vi "DI Scope Run.vi"(8 "error in":errorcluster, 11 "RT Data In":refnum<class "DCM-NIVS-RT.lvclass">) -> (0 "error out":errorcluster, 3 "RT Data Out":refnum<class "DCM-NIVS-RT.lvclass">)   [LabVIEW 2016, in "DCM Engine.lvlib"]
uses:
  DCM Engine.lvlib
  Classes/DCM-NIVS-RT/DCM-NIVS-RT.lvclass
  Classes/DCM-NIVS-RT/CompiledData Read.vi
  Classes/DCM-NIVS-RT/DCM Ref Read.vi
  Classes/DCM-NIVS-RT/Device Inputs Read.vi
  Classes/DCM-NIVS-RT/Device Outputs Read.vi
  Classes/DCM-NIVS-RT/CompiledData Write.vi
  Classes/DCM-NIVS-RT/Device Outputs Write.vi
  <vilib>/NI Veristand/Custom Device Waveform API/Multiple Waveforms Write (DBL)/Multiple Waveforms Write (DBL).lvclass
  Built/DCM Classes Packed/Pharlap/C/DCM-Classes.lvlibp/DCM/Rev0/RT/DCM - RT.lvclass
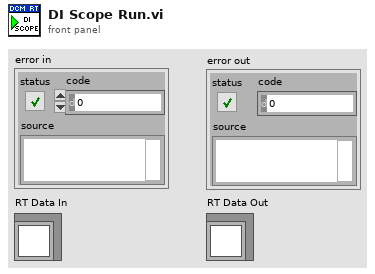
[diagram p1: front panel]
types:
  T1 = typedef "DCM Shared.lvlib/Compiled Data.ctl" = cluster{"Init":T2, "Cmd Status":T3, "Sys Status":T3, "EPTx RevA":T4, "DCM Core":T7, "DI-A Injection":T17, "DI-B Injection":T17, "DiffIO":T24, "HH Cmd":T27, "DI ADC":T29, "HH ADC":T31, "Digital Signals":T32, "Skip Fire":T33, "Knock":T35, "PBx":T36}
  T2 = typedef "DCM Shared.lvlib/Engine Init Data.ctl" = cluster{"Name":string, "RIO Address":string, "Bitfile Path RT":path, "Username":string, "Password":string, "Cmd CPU":i32, "Cmd Decimation":i32, "Cmd Priority":i32, "Sys CPU":i32, "Sys Decimation":i32, "Sys Priority":i32, "Input FIFO Size":i32, "Output FIFO Size":i32, "Compile Time":dbl}
  T3 = typedef "DCM Shared.lvlib/Engine Status.ctl" = cluster{"FIFO indexes":cluster{"code":i32, "loop duration":i32, "late count":i32}}
  T4 = typedef "DCM Shared.lvlib/EPTx RevA RT Data.ctl" = cluster{"FIFO Indexes":cluster{"Read":cluster{"Sync":i32, "CurrentCAD":i32, "Speed":i32, "Config":i32, "Rcvg Primary":i32, "Stall":i32, "Overflow Error":i32, "Ratio Error":i32, "Pattern Error":i32, "Aux Warning":i32, "Watchdog Error":i32, "Loading":i32}, "Write":cluster{"Reload EPTx":i32, "Sync Enable":i32, "Clear Errors":i32, "Sim Enable":i32, "Sim Speed":i32}}, "Settings":cluster{"EPTxConfigFilename":string, "EPTx Signal Select":cluster{"Primary":T5, "Aux 1":T5, "Aux 2":T5, "Aux 3":T5, "Aux 4":T5}, "FPGAFrequency":sgl, "StallSpeed":sgl, "EPTxFilters":T6, "History":u8}}
  T5 = typedef "DCM-Classes.lvlibp/DCM - FPGA.lvlib/Digital Channel.ctl" = enum8{"Unused", "User OS", "Diff IO 1", "Diff IO 2", "Diff IO 3", "Diff IO 4", "Diff IO 5", "Diff IO 6", "Diff IO 7", "Diff IO 8", "Aux 1", "Aux 2", "Aux 3", "Aux 4", "Aux 5", "Aux 6", "Aux 7", "Aux 8", "Aux 9", "Aux 10", "Aux 11", "Aux 12", "Aux 13", "Aux 14", "Aux 15", "Aux 16"}
  T6 = typedef "DCM-Classes.lvlibp/EPTx - RevA - RT.lvlib/EPTxFilters.ctl" = cluster{"Primary [s]":sgl, "Aux 1 [s]":sgl, "Aux 2 [s]":sgl, "Aux 3 [s]":sgl, "Aux 4 [s]":sgl}
  T7 = typedef "DCM Shared.lvlib/DCM Core.ctl" = cluster{"FIFO Indexes":cluster{"A Run State":i32, "B Run State":i32, "Read":cluster{"Status":T8, "A DI Faults":T9[], "B DI Faults":T9[], "HH Status":T10[]}, "Write":cluster{"A Config":cluster{"PowerSupplyEnable":i32, "InjectEnable":i32, "BoostVoltage":i32}, "B Config":cluster{"PowerSupplyEnable":i32, "InjectEnable":i32, "BoostVoltage":i32}, "HH Config":T11[], "System Settings":cluster{"MPRD":i32, "UserLED1":i32, "UserLED2":i32}, "A Fault Clear":cluster{"1":i32, "2":i32, "3":i32, "4":i32, "5":i32, "6":i32, "7":i32, "8":i32}, "B Fault Clear":cluster{"1":i32, "2":i32, "3":i32, "4":i32, "5":i32, "6":i32, "7":i32, "8":i32}}}, "Settings":cluster{"A Configuration":T12, "B Configuration":T12, "System Settings":T14}}
  T8 = typedef "DCM Shared.lvlib/System State Indexes.ctl" = cluster{"System ADC":cluster{"AI 1 [V]":i32, "AI 2 [V]":i32, "AI 3 [V]":i32, "AI 4 [V]":i32, "AI 5 [V]":i32, "AI 6 [V]":i32, "AI 7 [V]":i32, "AI 8 [V]":i32, "AI 9 [V]":i32, "AI 10 [V]":i32, "AI 11 [V]":i32, "AI 12 [V]":i32, "Temp HH 1-6 [C]":i32, "Temp HH 7-12 [C]":i32, "Temp DI A [C]":i32, "Temp DI Zener A [C]":i32, "Temp DI B [C]":i32, "Temp DI Zener B [C]":i32, "Temp CPU [C]":i32, "Temp Fan Intake [C]":i32, "Temp Secondary A [C]":i32, "Temp Primary A [C]":i32, "Temp Boost B [C]":i32, "Primary Range [V]":i32, "Primary A1A2 [V]":i32, "Primary A3A4 [V]":i32, "Primary B3B4 [V]":i32, "Primary B1B2 [V]":i32, "Secondary A1A2 [V]":i32, "Secondary A3A4 [V]":i32, "Secondary B3B4 [V]":i32, "Secondary B1B2 [V]":i32, "Ext HV A [V]":i32, "Ext HV B [V]":i32, "FET Driver [V]":i32, "Fan [V]":i32, "Battery [V]":i32, "DRVP [V]":i32, "Key [V]":i32, "DI Zener A [V]":i32, "DI Zener B [V]":i32, "Pump Zener A [V]":i32, "Pump Zener B [V]":i32, "MPRD [V]":i32}, "IO Lock":i32, "HH Mode Config Error":i32, "Fan Speed 1 [RPM]":i32, "Fan Speed 2 [RPM]":i32, "Firmware Major Rev":i32, "Firmware Minor Rev":i32, "Internal Fault":i32, "Fault Value":i32}
  T9 = typedef "DCM Shared.lvlib/DI Faults Indexes.ctl" = cluster{"HV Fault":i32, "LV Fault":i32, "LS Fault":i32, "MUX Fault":i32, "Open Warning":i32}
  T10 = typedef "DCM Shared.lvlib/HH Status Indexes.ctl" = cluster{"Current [A]":i32, "Config Error":i32, "Short Fault":i32, "Open Fault":i32, "Period Min [A]":i32, "Period Max [A]":i32, "Period Avg [A]":i32, "On Avg [A]":i32}
  T11 = typedef "DCM Shared.lvlib/HH Config Indexes.ctl" = cluster{"Mode":i32, "IO Lock State":i32, "Phase 1 FP":i32, "Fault Clear":i32, "ISeq":cluster{"Upper [A]":i32, "Lower [A]":i32, "Duration [s]":i32}[]}
  T12 = typedef "DCM - RT.lvclass/Configuration.ctl" = cluster{"Configuration":T13, "Power Supply Enable":bool, "Boost Voltage [V]":sgl, "Inject Enable":bool, "DI Zener Enable":bool, "DI Zener Voltage [V]":sgl, "Pump Zener Enable":bool, "Pump Zener Voltage [V]":sgl, "Boost Clamp [V]":sgl}
  T13 = typedef "DCM - FPGA.lvlib/DI - Bank Configuration.ctl" = enum8{"Solenoid Unipolar 4", "Solenoid Unipolar 7 (Muxed)", "Solenoid Unipolar 8 (Muxed)", "Solenoid Bipolar 2", "Solenoid Bipolar 3 (Muxed)", "Piezo Unipolar 2", "Piezo Unipolar 3 (Muxed)", "Piezo Unipolar 4 (Muxed)", "Piezo Bipolar 2", "Piezo Bipolar 3 (Muxed)"}
  T14 = typedef "DCM - RT.lvclass/System Settings.ctl" = cluster{"MPRD":bool, "IO Lock MPRD Disable":bool, "User LED 1":T15, "User LED 2":T15, "DI HS Fault Filter Time [s]":sgl, "Clamp Fault Filter Time [s]":sgl, "HH Shoot Through Time [s]":sgl, "HH ISeq Dur PS":T16, "HH Open Threshold [A]":sgl}
  T15 = typedef "DCM - RT.lvclass/User LED.ctl" = enum16{"Off", "Yellow", "Green"}
  T16 = typedef "DCM - RT - HH.lvlib/Duration Pre Scale.ctl" = u8
  T17 = typedef "DCM Shared.lvlib/DI.ctl" = cluster{"DI Command Enabled":bool, "Sync Pump Enabled":bool, "FIFO Indexes":cluster{"Write":cluster{"DI Command":T18[], "Pump Command":T18}}, "Settings":T19}
  T18 = typedef "DCM Shared.lvlib/DI Command Indexes.ctl" = cluster{"Mode":i32, "Digital Input":i32, "Default Profile Index":i32, "Cal Freq [Hz]":i32, "Cal Duration [s]":i32, "Cal Increment [s]":i32, "Cal Pulses":i32, "TMP Command Sequence":cluster{"Duration [s]":i32, "Level":i32, "Run/Stop":i32, "Profile Index":i32}[], "EPT TDC Offset [CAD]":i32, "EPT Window Start [DBTDC]":i32, "EPT Window End [DBTDC]":i32, "EPT Angles":cluster{"Enable":i32, "Timing [DBTDC]":i32, "Duration [s]":i32, "Profile Index":i32}[], "EPT Skip Fire":i32, "EPT Skip Index":i32, "EPT Precharge Duration [s]":i32, "EPT Precharge Profile Index":i32}
  T19 = typedef "DCM Shared.lvlib/DI Phase Outputs.ctl" = cluster{"Inj Phase Arrays":T20[][], "Pump Phase Array":T20[], "Pulsewidths [s]":sgl[][]}
  T20 = typedef "DCM - RT - DI.lvlib/Phase.ctl" = cluster{"Drive":T21, "Direction":bool, "Phase Step":T22, "Duration [s]":sgl, "Current High [A]":sgl, "Current Low [A]":sgl, "Voltage High [V]":sgl, "Voltage Low [V]":sgl, "Change":bool, "Current Control":T23, "Period [s]":sgl, "Pulse Width [s]":sgl, "Profile":u8, "Voltage Control":bool}
  T21 = typedef "DCM - FPGA.lvlib/DI - Drive State.ctl" = enum8{"Idle", "HV Current Control", "LV Current Control", "Back Boost", "Piezo Charge", "Piezo Discharge"}
  T22 = typedef "DCM - FPGA - DI.lvlib/Phase Step.ctl" = enum8{"Duration", "First Peak", "End of Cmd", "Branch", "2-Phase Duration"}
  T23 = typedef "DCM - FPGA - DI.lvlib/Control.ctl" = enum8{"Closed Loop", "Fixed Period", "Fixed On Pulse", "Fixed Off Pulse", "Open Loop", "Profile"}
  T24 = typedef "DCM Shared.lvlib/DiffIO.ctl" = cluster{"DiffIO Command Enabled":bool, "FIFO Indexes":cluster{"Read":cluster{"Diff IO Results":T25[], "DiffIOIn":cluster{"1":i32, "2":i32, "3":i32, "4":i32, "5":i32, "6":i32, "7":i32, "8":i32}}, "Write":cluster{"Diff I/O Setup":T26[]}}}
  T25 = typedef "DCM Shared.lvlib/DiffIO Results Indexes.ctl" = cluster{"Capture [DBTDC]":i32, "Capture Error":i32, "Frequency [Hz]":i32, "Duty Cycle [%]":i32, "PWM Stopped":i32}
  T26 = typedef "DCM Shared.lvlib/DiffIO Setup Indexes.ctl" = cluster{"Mode":i32, "Capture Start [DBTDC]":i32, "Capture End [DBTDC]":i32, "Invert":i32, "Frequency [Hz]":i32, "Duty Cycle [%]":i32, "TDC Offset [CAD]":i32, "Window Start [DBTDC]":i32, "Window End [DBTDC]":i32, "Angles":cluster{"Enable":i32, "Location [DBTDC]":i32, "Duration [s]":i32}[], "Skip Fire":i32, "Skip Fire Index":i32}
  T27 = typedef "DCM Shared.lvlib/HH.ctl" = cluster{"HH Command Enabled":bool, "FIFO Indexes":cluster{"Write":T28[]}}
  T28 = typedef "DCM Shared.lvlib/HH Command Indexes.ctl" = cluster{"Mode":i32, "Digital Input":i32, "Polarity":i32, "Frequency [Hz]":i32, "Duty Cycle [%]":i32, "TDC Offset [CAD]":i32, "Window Start [DBTDC]":i32, "Window End [DBTDC]":i32, "Angles":cluster{"Enable":i32, "Location [DBTDC]":i32, "Duration [s]":i32}[], "Skip Fire":i32, "Skip Fire Index":i32}
  T29 = typedef "DCM Shared.lvlib/DI Scope.ctl" = cluster{"FIFO Indexes":cluster{"Write":cluster{"Capture Enable":i32, "Capture Event":i32, "Capture Length":i32, "DI ADC 1 Select":i32, "DI ADC 2 Select":i32, "DI ADC 3 Select":i32, "DI ADC 4 Select":i32}, "Read":cluster{"Capture dt [s]":i32}}, "DI ADC Data":cluster{"Output Array":sgl[][], "New Data":bool}, "Waveform Data":T30[], "Waveform Session":refnum<class "Multiple Waveforms Write (DBL).lvclass">}
  T30 = typedef "Custom Device API.lvlib/Waveform Data Reference.ctl" = i32
  T31 = typedef "DCM Shared.lvlib/HH Scope.ctl" = cluster{"FIFO Indexes":cluster{"Write":cluster{"Capture Enable":i32, "Capture Event":i32, "Capture Length":i32}, "Read":cluster{"Capture dt [s]":i32}}, "HH ADC Data":cluster{"Output Array":sgl[][], "New Data":bool}, "Waveform Data":T30[], "Waveform Session":refnum<class "Multiple Waveforms Write (DBL).lvclass">}
  T32 = typedef "DCM Shared.lvlib/Digital Signals.ctl" = cluster{"FIFO Indexes":cluster{"Write":cluster{"User OS":i32, "User OS Time [s]":i32}}, "Settings":cluster{"Diff IO Filters [s]":sgl[], "Aux In Filters [s]":sgl[], "Serial In 1":T5, "Serial In 2":T5}}
  T33 = typedef "DCM Shared.lvlib/Skip Fire.ctl" = cluster{"Skip Fire Enabled":bool, "FIFO Indexes":cluster{"Write":cluster{"Setup":T34[]}}}
  T34 = typedef "DCM Shared.lvlib/Skip Fire Setup Indexes.ctl" = cluster{"Enable":i32, "Total Cycles":i32, "On Cycles":i32, "TDC Offset [CAD]":i32}
  T35 = typedef "DCM Shared.lvlib/Knock.ctl" = cluster{"Knock Enabled":bool, "FIFO Indexes":cluster{"Read":cluster{"Knock":i32[], "Knock Intensity":i32[]}, "Write":cluster{"Low Cutoff [Hz]":i32, "High Cutoff [Hz]":i32, "Threshold":i32, "Knock Start [CAD]":i32, "Knock End [CAD]":i32, "Reference Start [CAD]":i32, "Reference End [CAD]":i32}}, "Settings":cluster{"Sensor Select":i32[], "Cylinder Offset [CAD]":sgl[]}}
  T36 = typedef "DCM Shared.lvlib/PBx.ctl" = cluster{"PB Version":u8, "PB-01":T37}
  T37 = typedef "DCM Shared.lvlib/PB-01.ctl" = cluster{"FIFO Indexes":cluster{"Write":cluster{"Clear Faults":i32, "ESTTL Setup":T38[], "UEGO Control":cluster{"UEGO1Enable":i32, "UEGO2Enable":i32, "UEGO1Range":i32, "UEGO2Range":i32, "FilterCutoff (Hz)":i32}}, "Read":cluster{"UEGO Sensor Results":cluster{"UEGO1Lambda":i32, "UEGO1Phi":i32, "UEGO1AFRatio":i32, "UEGO1Ip (mA)":i32, "UEGO2Lambda":i32, "UEGO2Phi":i32, "UEGO2AFRatio":i32, "UEGO2Ip (mA)":i32}, "UEGO Temperature (C)":cluster{"UEGO1Temp (C)":i32, "UEGO2Temp (C)":i32, "UEGO1Hot":i32, "UEGO2Hot":i32}, "UEGO Diagnostics":cluster{"UEGO1SensorFault":i32, "UEGO2SensorFault":i32, "UEGO1HeaterFault":i32, "UEGO2HeaterFault":i32, "UEGOFuseStatus":i32, "Battery (V)":i32, "LSUType":i32}}}, "Settings":cluster{"VR-Hall Mode Select":T39[], "VR-Hall Arming Threshold [V]":dbl[], "ESTTL Command Enabled":bool}}
  T38 = typedef "DCM Shared.lvlib/ESTTL Setup Indexes.ctl" = cluster{"Mode":i32, "Polarity":i32, "Frequency [Hz]":i32, "Duty Cycle [%]":i32, "TDC Offset [CAD]":i32, "Window Start [DBTDC]":i32, "Window End [DBTDC]":i32, "Angles":cluster{"Enable":i32, "Location [DBTDC]":i32, "Duration [s]":i32}[], "Skip Fire":i32, "Skip Fire Index":i32}
  T39 = typedef "Vr_Hall_mode_control_revc.ctl" = enum32{"VR Adaptive Arm", "VR Manual Arm", "Hall", "Hall w/ Pull-up"}
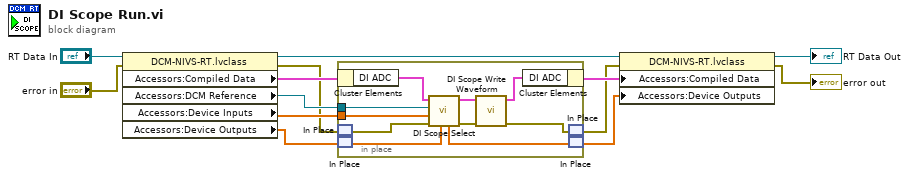
[diagram p0: block diagram]
diagram:
  n1 = property class="DCM-NIVS-RT.lvclass"(reference="RT Data In", error in="error in") -> (reference out=w9:refnum<class "DCM-NIVS-RT.lvclass">, error out=w4:errorcluster, "Accessors:Compiled Data"=w8:T1, "Accessors:DCM Reference"=w12:refnum<class "DCM - RT.lvclass">, "Accessors:Device Inputs"=w13:dbl[], "Accessors:Device Outputs"=w2:dbl[])
  n2 = in-place {
    in-place-border: w13 -> [w23]
    in-place-border: w12 -> [w21]
    n3 = in-place-cluster #1(w8) -> ("DI ADC"=w19:T29)
    n4 = in-place-match #2(w4) -> (w17:errorcluster)
    n5 = in-place-match #3(w2) -> (w15:dbl[])
    n6 = call "DI Scope Select.vi"("Device Outputs in"=w15, "error in"=w17, "Device Inputs"=w23, "DCM Ref"=w21, "DI ADC in"=w19) -> ("error out"=w22:errorcluster, "DI ADC out"=w20:T29, "Device Outputs out"=w14:dbl[])  [unwired: 4 in]
    n7 = call "DI Scope Write Waveform.vi"("error in"=w22, "DI ADC in"=w20) -> ("error out"=w16:errorcluster, "DI ADC out"=w18:T29)  [unwired: 8 in]
    n8 = in-place-cluster #1("DI ADC"=w18) -> (w7:T1)
    n9 = in-place-match #2(w16) -> (w3:errorcluster)
    n10 = in-place-match #3(w14) -> (w1:dbl[])
  }
  n11 = property class="DCM-NIVS-RT.lvclass"(reference=w9, error in=w3, "Accessors:Compiled Data"=w7, "Accessors:Device Outputs"=w1) -> (reference out=→"RT Data Out":refnum<class "DCM-NIVS-RT.lvclass">, error out=→"error out":errorcluster)
